vi "Set UI VI Ref (nonreplacing).vi"(8 "error in (no error)":errorcluster, 10 "UI VI Ref":refnum<vi>, 11 "ViewableActor in":refnum<class "ViewableActor.lvclass">) -> (0 "error out":errorcluster, 1 "Top Level UI?":bool, 3 "ViewableActor out":refnum<class "ViewableActor.lvclass">)   [LabVIEW 2012, in "Win8uiFramework.lvlib" / "ViewableActor.lvclass"]
uses:
  ViewableActor.lvclass
  ViewableActor.lvclass/ViewableActor.ctl
  Write UI VI Ref.vi
  Read UI VI Ref.vi
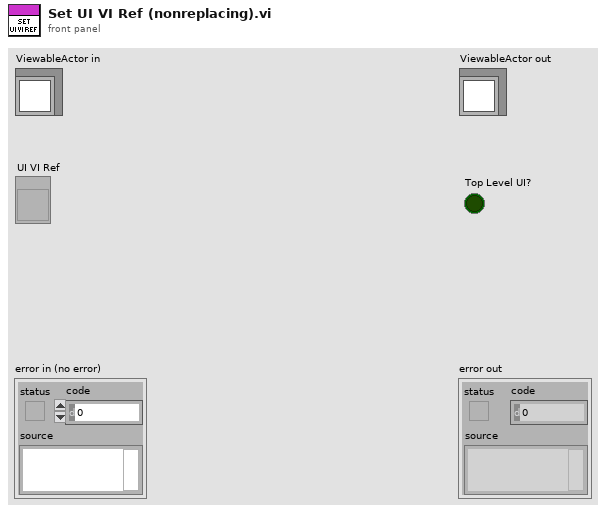
[diagram p1: front panel]
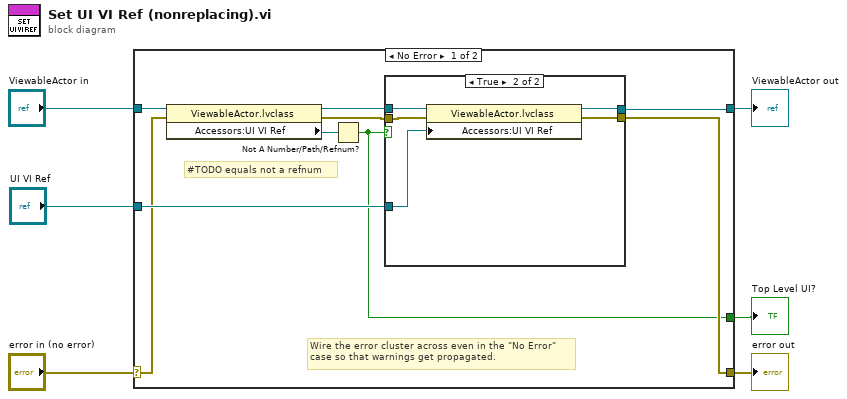
[diagram p0: block diagram]
diagram:
  n1 = case shown="No Error" "error in (no error)" {
    selector: "error in (no error)" -> [w10 w24]
    tunnel: [w8 w24] -> w5
    tunnel: [w12 w23] -> w3
    tunnel: "ViewableActor in" -> [w15 w23]
    tunnel: "UI VI Ref" -> [w11 _]
    tunnel: [w7 _] -> w1
    frame No Error {
      # "#TODO equals not a refnum"
      # "Wire the error cluster across even in the \"No Error\"\ncase so that warnings get propagated."
      n2 = property class="ViewableActor.lvclass"(reference=w15, error in=w10) -> (reference out=w13:refnum<class "ViewableActor.lvclass">, error out=w9:errorcluster, "Accessors:UI VI Ref"=w14:refnum<vi>)
      n3 = Not A Number/Path/Refnum?(number/path/refnum=w14) -> (NaN/Path/Refnum?=w7:bool)
      n4 = case shown="True" w7 {
        tunnel: w13 -> [w17 w22]
        tunnel: [w17 w21] -> w12
        tunnel: w11 -> [_ w20]
        tunnel: w9 -> [w16 w19]
        tunnel: [w16 w18] -> w8
        frame False {
        }
        frame True {
          n5 = property class="ViewableActor.lvclass"(reference=w22, error in=w19, "Accessors:UI VI Ref"=w20) -> (reference out=w21:refnum<class "ViewableActor.lvclass">, error out=w18:errorcluster)
        }
      }
    }
    frame Error {
    }
  }
  "error out" <- w5
  "ViewableActor out" <- w3
  "Top Level UI?" <- w1
